vi "Create Down Templates.vi"   [LabVIEW 2014]
uses:
  <vilib>/vision/NI_Vision_Development_Module.lvlib
types:
  T1 = typedef "Image Type" = u32
  T2 = typedef "IMAQ Image.ctl" = refnum<image>
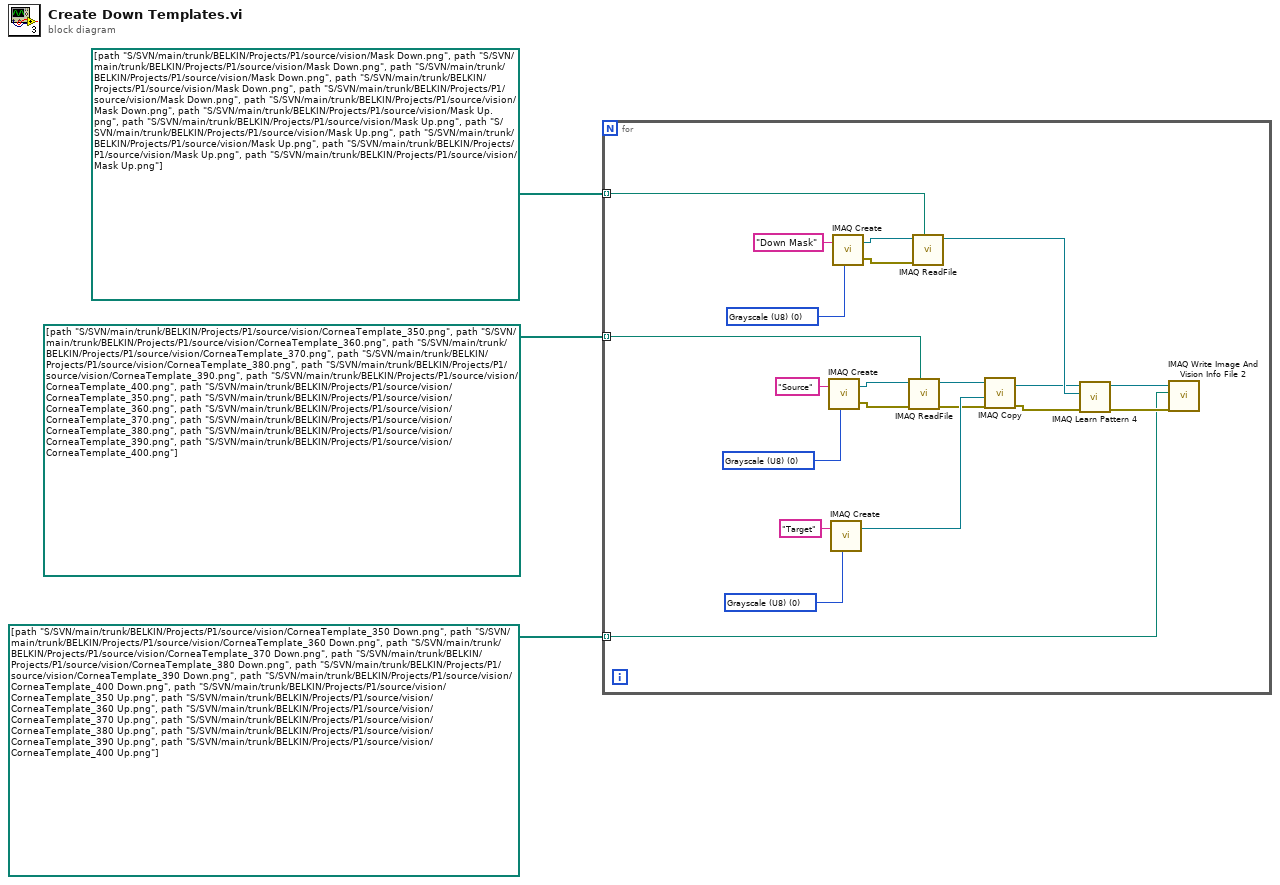
[diagram p0: block diagram]
diagram:
  n1 = for {
    tunnel: path[] [path "S:/SVN/main/trunk/BELKIN/Projects/P1/source/vision/Mask Down.png", path "S:/SVN/main/trunk/BELKIN/Projects/P1/source/vision/Mask Down.png", path "S:/SVN/main/trunk/BELKIN/Projects/P1/source/vision/Mask Down.png", path "S:/SVN/main/trunk/BELKIN/Projects/P1/source/vision/Mask Down.png", path "S:/SVN/main/trunk/BELKIN/Projects/P1/source/vision/Mask Down.png", path "S:/SVN/main/trunk/BELKIN/Projects/P1/source/vision/Mask Down.png", path "S:/SVN/main/trunk/BELKIN/Projects/P1/source/vision/Mask Up.png", path "S:/SVN/main/trunk/BELKIN/Projects/P1/source/vision/Mask Up.png", path "S:/SVN/main/trunk/BELKIN/Projects/P1/source/vision/Mask Up.png", path "S:/SVN/main/trunk/BELKIN/Projects/P1/source/vision/Mask Up.png", path "S:/SVN/main/trunk/BELKIN/Projects/P1/source/vision/Mask Up.png", path "S:/SVN/main/trunk/BELKIN/Projects/P1/source/vision/Mask Up.png"] -> [w20] mode=indexing
    tunnel: path[] [path "S:/SVN/main/trunk/BELKIN/Projects/P1/source/vision/CorneaTemplate_350.png", path "S:/SVN/main/trunk/BELKIN/Projects/P1/source/vision/CorneaTemplate_360.png", path "S:/SVN/main/trunk/BELKIN/Projects/P1/source/vision/CorneaTemplate_370.png", path "S:/SVN/main/trunk/BELKIN/Projects/P1/source/vision/CorneaTemplate_380.png", path "S:/SVN/main/trunk/BELKIN/Projects/P1/source/vision/CorneaTemplate_390.png", path "S:/SVN/main/trunk/BELKIN/Projects/P1/source/vision/CorneaTemplate_400.png", path "S:/SVN/main/trunk/BELKIN/Projects/P1/source/vision/CorneaTemplate_350.png", path "S:/SVN/main/trunk/BELKIN/Projects/P1/source/vision/CorneaTemplate_360.png", path "S:/SVN/main/trunk/BELKIN/Projects/P1/source/vision/CorneaTemplate_370.png", path "S:/SVN/main/trunk/BELKIN/Projects/P1/source/vision/CorneaTemplate_380.png", path "S:/SVN/main/trunk/BELKIN/Projects/P1/source/vision/CorneaTemplate_390.png", path "S:/SVN/main/trunk/BELKIN/Projects/P1/source/vision/CorneaTemplate_400.png"] -> [w19] mode=indexing
    tunnel: path[] [path "S:/SVN/main/trunk/BELKIN/Projects/P1/source/vision/CorneaTemplate_350 Down.png", path "S:/SVN/main/trunk/BELKIN/Projects/P1/source/vision/CorneaTemplate_360 Down.png", path "S:/SVN/main/trunk/BELKIN/Projects/P1/source/vision/CorneaTemplate_370 Down.png", path "S:/SVN/main/trunk/BELKIN/Projects/P1/source/vision/CorneaTemplate_380 Down.png", path "S:/SVN/main/trunk/BELKIN/Projects/P1/source/vision/CorneaTemplate_390 Down.png", path "S:/SVN/main/trunk/BELKIN/Projects/P1/source/vision/CorneaTemplate_400 Down.png", path "S:/SVN/main/trunk/BELKIN/Projects/P1/source/vision/CorneaTemplate_350 Up.png", path "S:/SVN/main/trunk/BELKIN/Projects/P1/source/vision/CorneaTemplate_360 Up.png", path "S:/SVN/main/trunk/BELKIN/Projects/P1/source/vision/CorneaTemplate_370 Up.png", path "S:/SVN/main/trunk/BELKIN/Projects/P1/source/vision/CorneaTemplate_380 Up.png", path "S:/SVN/main/trunk/BELKIN/Projects/P1/source/vision/CorneaTemplate_390 Up.png", path "S:/SVN/main/trunk/BELKIN/Projects/P1/source/vision/CorneaTemplate_400 Up.png"] -> [w4] mode=indexing
    w14 = T1 0 items=["Grayscale (U8)", "Grayscale (I16)", "Grayscale (SGL)", "Complex (CSG)", "RGB (U32)", "HSL (U32)", "RGB (U64)", "Grayscale (U16)"] ("Image Type")
    w15 = T1 0 items=["Grayscale (U8)", "Grayscale (I16)", "Grayscale (SGL)", "Complex (CSG)", "RGB (U32)", "HSL (U32)", "RGB (U64)", "Grayscale (U16)"] ("Image Type")
    w24 = T1 0 items=["Grayscale (U8)", "Grayscale (I16)", "Grayscale (SGL)", "Complex (CSG)", "RGB (U32)", "HSL (U32)", "RGB (U64)", "Grayscale (U16)"] ("Image Type")
    n2 = call "IMAQ Create"("Image Name"="Source", "Image Type"=w15) -> ("New Image"=w17:T2, "error out"=w18:errorcluster)  [unwired: 3 in]
    n3 = call "IMAQ Create"("Image Name"="Target", "Image Type"=w14) -> ("New Image"=w10:T2)  [unwired: 3 in, 1 out]
    n4 = call "IMAQ Create"("Image Name"="Down Mask", "Image Type"=w24) -> ("New Image"=w22:T2, "error out"=w21:errorcluster)  [unwired: 3 in]
    n5 = call "IMAQ ReadFile"("File Path"=w19, "error in (no error)"=w18, "Image"=w17) -> ("error out"=w7:errorcluster, "Image Out"=w11:T2)  [unwired: 4 in, 3 out]
    n6 = call "IMAQ ReadFile"("File Path"=w20, "error in (no error)"=w21, "Image"=w22) -> ("Image Out"=w12:T2)  [unwired: 4 in, 4 out]
    n7 = call "IMAQ Copy"("error in (no error)"=w7, "Image Dst"=w10, "Image Src"=w11) -> ("error out"=w6:errorcluster, "Image Dst Out"=w9:T2)  [unwired: 3 in]
    n8 = call "IMAQ Learn Pattern 4"("error in (no error)"=w6, "Mask"=w12, "Image"=w9) -> ("error out"=w5:errorcluster, "Template Image Out"=w8:T2)  [unwired: 6 in, 1 out]
    n9 = call "IMAQ Write Image And Vision Info File 2"("error in (no error)"=w5, "File Path"=w4, "Image"=w8) -> ()  [unwired: 7 in, 2 out]
  }
